vi "niusrprios DDC (Multi-Channel).vi"(0 "data in":T1[](array[typedef])=[{"I"=0.0, "Q"=0.0, "overflow"=FALSE}, {"I"=0.0, "Q"=0.0, "overflow"=FALSE}], 1 "reset":bool, 5 "start trigger":bool, 9 "enabled":bool[](array[boolean])=[FALSE, FALSE], 11 "DDC Parameters":T2[](array[typedef])=[{"output sample rate"=0.0, "delay"=0.0, "frequency shift"=0.0, "impairments"={"inline gain I"=0.0, "inline gain Q"=0.0, "cross gain I"=0.0, "cross gain Q"=0.0, "pre-gain offset I"=0.0, "pre-gain offset Q"=0.0, "post-gain offset I"=0.0, "post-gain offset Q"=0.0}, "phase"=0.0}, {"output sample rate"=0.0, "delay"=0.0, "frequency shift"=0.0, "impairments"={"inline gain I"=0.0, "inline gain Q"=0.0, "cross gain I"=0.0, "cross gain Q"=0.0, "pre-gain offset I"=0.0, "pre-gain offset Q"=0.0, "post-gain offset I"=0.0, "post-gain offset Q"=0.0}, "phase"=0.0}] {"frequency shift" format="%#.48g"}) -> (4 "data out":u32[](array[numeric]), 6 "number of overflows":u64[](array[numeric]), 10 "output valid":bool, 14 "dsp reset done":bool)   [LabVIEW 2015]
doc: "Digital downconverter (DDC) for two channels which can be extended to more channels. Implemented with FPGA-based DSP.\n\n<B>Input Parameters</B>\n\n<B>data in</B> is the I and Q data to be downconverted along with overflow information.\n\n<B>start trigger</B> triggers the Rx signal chain if an Rx stream is enabled.\n\n<B>enabled</B> specifies which streams are enabled.\n\n<B>DDC Parameters</B> are the downconversion parameters utilized by the DSP chain.\n\n<B>reset</B> the DSP downconversion signal chain.\n\n<B>Output Parameters</B>\n\n<B>dsp reset done</B> indicates that the DSP downconversion signal chain completed reset.\n\n<B>data out</B> is the downconverted data.\n\n<B>number of overflows</B> is the number of times the DSP chain overflowed on fixed point conversion of 'data in'.\n\n<B>output valid</B> specifies when 'data out' is valid."
uses:
  niusrprios DDC Parameters.ctl
  <instrlib>/_niInstr/DSP/v1/Shared/Public/IQ Impairments.ctl
  <instrlib>/_niInstr/DSP/v1/Shared/Public/IQ Data.ctl
  <instrlib>/_niInstr/DSP/v1/Shared/niInstr DSP v1 Shared.lvlib
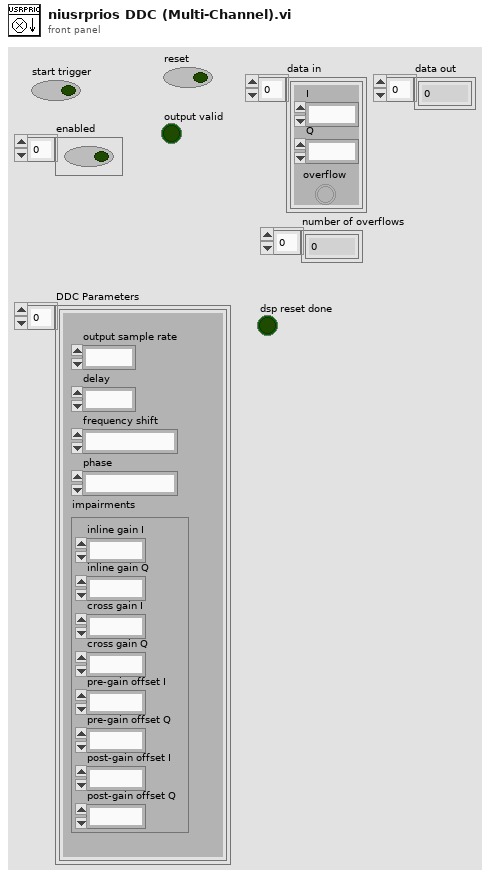
[diagram p1: front panel]
types:
  T1 = typedef "niInstr DSP v1 Shared.lvlib/IQ Data.ctl" = cluster{"I":fxp<+/-,18,1>, "Q":fxp<+/-,18,1>, "overflow":bool}
  T2 = typedef "niusrprios DDC Parameters.ctl" = cluster{"output sample rate":fxp<+,48,1>, "delay":fxp<+/-,16,0>, "frequency shift":fxp<+/-,48,0>, "impairments":T3, "phase":fxp<+/-,21,0>}
  T3 = typedef "niInstr DSP v1 Shared.lvlib/IQ Impairments.ctl" = cluster{"inline gain I":fxp<+/-,18,1>, "inline gain Q":fxp<+/-,18,1>, "cross gain I":fxp<+/-,18,1>, "cross gain Q":fxp<+/-,18,1>, "pre-gain offset I":fxp<+/-,18,1>, "pre-gain offset Q":fxp<+/-,18,1>, "post-gain offset I":fxp<+/-,18,1>, "post-gain offset Q":fxp<+/-,18,1>}
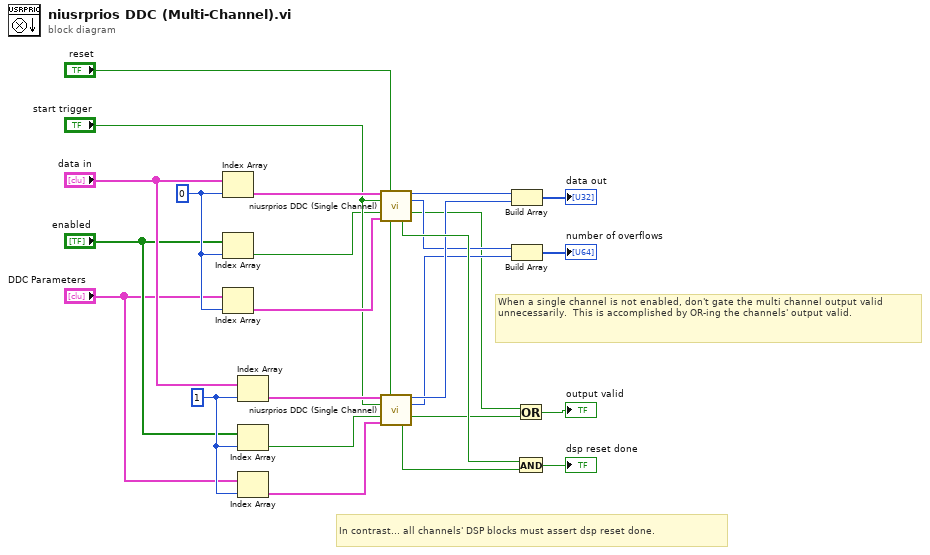
[diagram p0: block diagram]
diagram:
  w22 = 1 ("index")
  w23 = 0 ("index")
  # "When a single channel is not enabled, don't gate the multi channel output valid unnecessarily.  This is accomplished by OR-ing the channels' output valid."
  # "In contrast... all channels' DSP blocks must assert dsp reset done."
  n1 = Index Array(array="data in", index=w23) -> (element=w25:T1)
  n2 = Index Array(array="enabled", index=w23) -> (element=w4:bool)
  n3 = Index Array(array="DDC Parameters", index=w23) -> (element=w24:T2)
  n4 = Index Array(array="data in", index=w22) -> (element=w18:T1)
  n5 = Index Array(array="enabled", index=w22) -> (element=w3:bool)
  n6 = Index Array(array="DDC Parameters", index=w22) -> (element=w17:T2)
  n7 = call "niusrprios DDC (Single Channel).vi"("data in"=w25, "reset"="reset", "start trigger"="start trigger", "enabled"=w4, "DDC Parameters"=w24) -> ("data out"=w10:u32, "number of overflows"=w7:u64, "output valid"=w1:bool, "dsp reset done"=w14:bool)  [unwired: 7 in]
  n8 = call "niusrprios DDC (Single Channel).vi"("data in"=w18, "reset"="reset", "start trigger"="start trigger", "enabled"=w3, "DDC Parameters"=w17) -> ("data out"=w8:u32, "number of overflows"=w6:u64, "output valid"=w2:bool, "dsp reset done"=w13:bool)  [unwired: 7 in]
  n9 = Build Array(w10, w8) -> (→"data out":u32[])
  n10 = Build Array(w7, w6) -> (→"number of overflows":u64[])
  n11 = Or(x=w1, y=w2) -> (x .or. y?=→"output valid":bool)
  n12 = And(x=w14, y=w13) -> (x .and. y?=→"dsp reset done":bool)
